vi "GetValue.vi"(0 "reference":refnum<vi>, 1 "Input":string, 3 "error in (no error)":errorcluster) -> (7 "Answer":string, 9 "Found?":bool, 10 "error out":errorcluster)   [LabVIEW 2019]
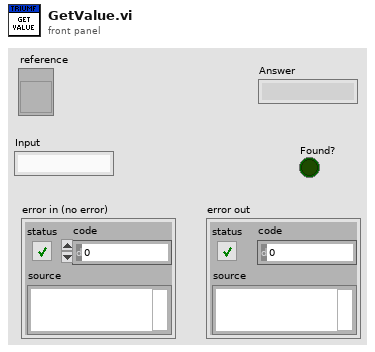
[diagram p1: front panel]
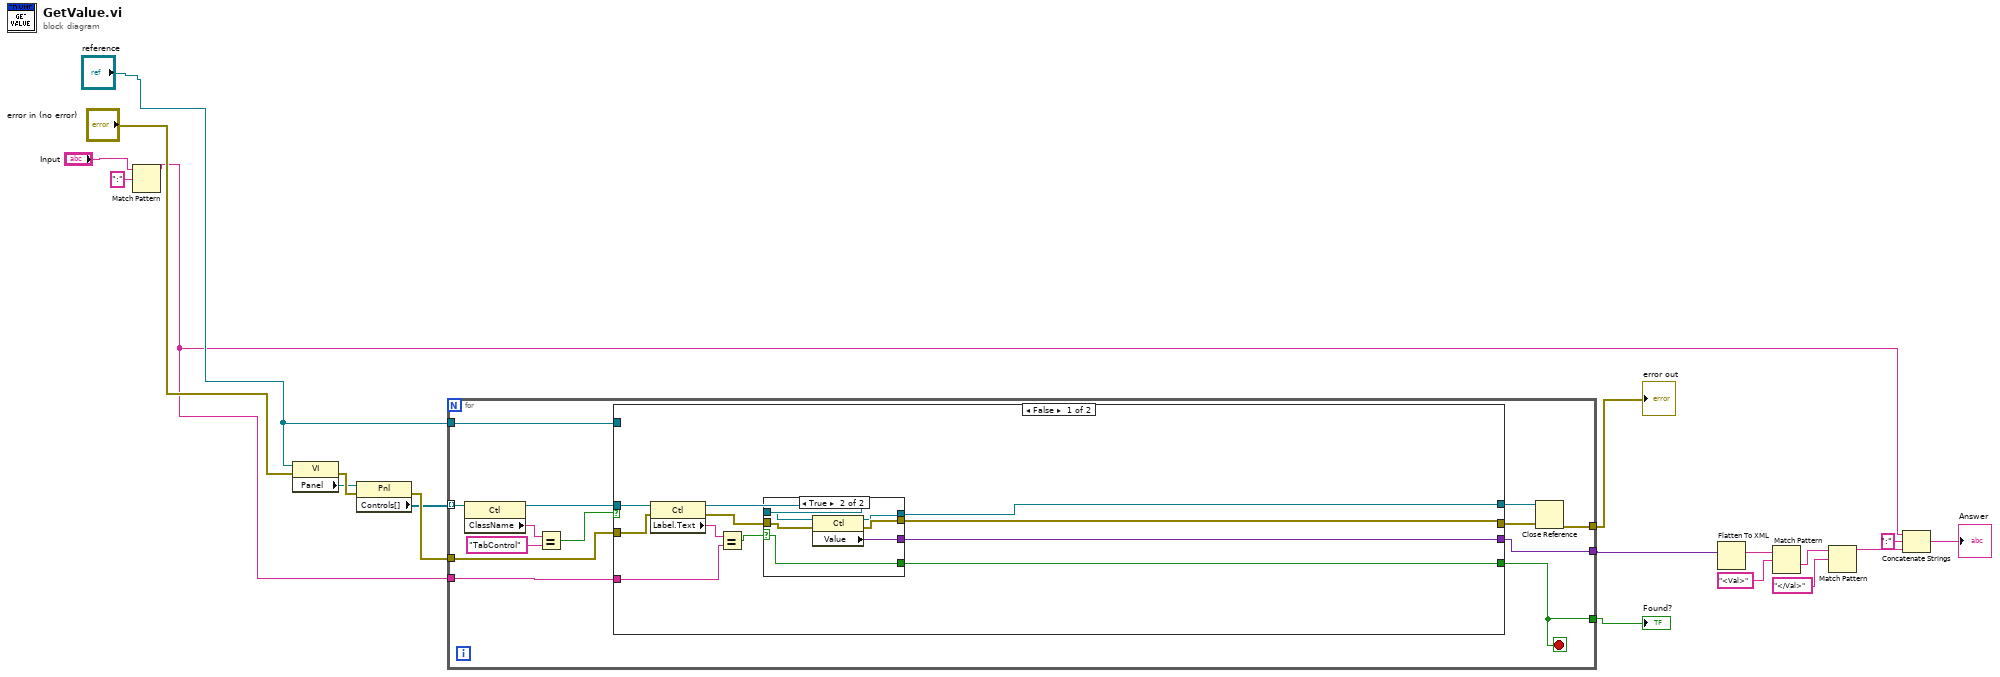
[diagram p0: block diagram]
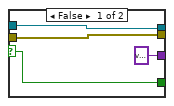
[diagram p2: hidden frame]
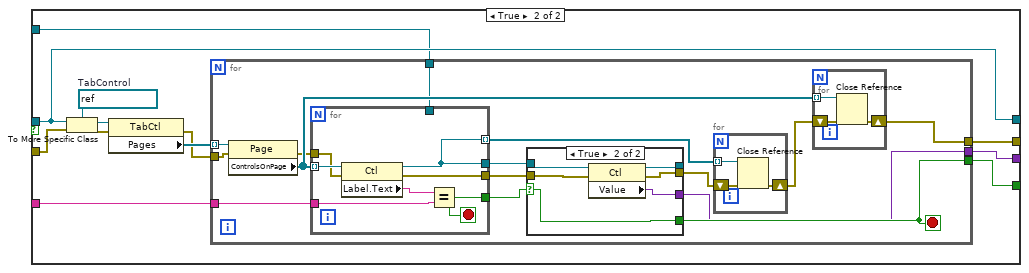
[diagram p3: hidden frame]
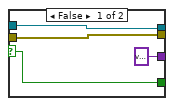
[diagram p4: hidden frame]
diagram:
  n1 = Match Pattern(string="Input", regular expression=":") -> (before substring=w1:string)  [unwired: 1 in, 3 out]
  n2 = property class="VI"(reference="reference", error in="error in (no error)") -> (error out=w14:errorcluster, "Panel"=w13:refnum<vi>)  [unwired: 1 out]
  n3 = property class="Pnl"(reference=w13, error in=w14) -> (error out=w15:errorcluster, "Controls[]"=w12:refnum<vi>[])  [unwired: 1 out]
  n4 = for {
    tunnel: w12 -> [w32] mode=indexing
    tunnel: "reference" -> [w25]
    tunnel: [w26] -> w10
    tunnel: w15 -> [w24]
    tunnel: w1 -> [w22]
    tunnel: [w21] -> w11
    tunnel: [w20] -> w3
    stop <- w21 stop-if-true
    n5 = property class="Ctl"(reference=w32) -> (reference out=w30:refnum<vi>, "ClassName"=w23:string)  [unwired: 1 in, 1 out]
    n6 = Equal?(x=w23, y="TabControl") -> (x = y?=w29:bool)
    n7 = case shown="False" w29 {
      tunnel: w30 -> [w43 w61]
      tunnel: [w35 w62] -> w28
      tunnel: [w36 w61] -> w27
      tunnel: w25 -> [_ w60]
      tunnel: w24 -> [w42 w59]
      tunnel: w22 -> [w40 w56]
      tunnel: [w34 w55] -> w21
      tunnel: [w33 w54] -> w20
      frame False {
        n8 = property class="Ctl"(reference=w43, error in=w42) -> (reference out=w37:refnum<vi>, error out=w38:errorcluster, "Label.Text"=w41:string)
        n9 = Equal?(x=w41, y=w40) -> (x = y?=w39:bool)
        n10 = case shown="True" w39 {
          selector: w39 -> [w45 w53]
          tunnel: [w47 w48] -> w36
          tunnel: w37 -> [w47 w52]
          tunnel: w38 -> [w46 w51]
          tunnel: [w46 w49] -> w35
          tunnel: [w45 w53] -> w34
          tunnel: [variant ("Value") w50] -> w33
          frame False {
          }
          frame True {
            n11 = property class="Ctl"(reference=w52, error in=w51) -> (reference out=w48:refnum<vi>, error out=w49:errorcluster, "Value"=w50:variant)
          }
        }
      }
      frame True {
        w64 = refnum<vi> refnum  # TabControl
        n12 = To More Specific Class(target class=w64, reference=w61, error in=w59) -> (specific class reference=w65:refnum<vi>, error out=w58:errorcluster)
        n13 = property class="TabCtl"(reference=w65, error in=w58) -> (error out=w57:errorcluster, "Pages"=w63:refnum<vi>[])  [unwired: 1 out]
        n14 = for {
          tunnel: w63 -> [w80] mode=indexing
          tunnel: [w78] -> w62
          tunnel: w60 -> [w77]
          tunnel: w57 -> [w76]
          tunnel: w56 -> [w74]
          tunnel: [w70] -> w55
          tunnel: [w66] -> w54
          stop <- w70 stop-if-true
          n15 = property class="Page"(reference=w80, error in=w76) -> (error out=w75:errorcluster, "ControlsOnPage"=w79:refnum<vi>[])  [unwired: 1 out]
          n16 = for {
            tunnel: w79 -> [w103] mode=indexing
            tunnel: [w98] -> w72
            tunnel: w77 -> [_]
            tunnel: w75 -> [w102]
            tunnel: w74 -> [w100]
            tunnel: [w99] -> w71
            tunnel: [w97] -> w69 mode=indexing
            tunnel: [w97] -> w73
            stop <- w99 stop-if-true
            n17 = property class="Ctl"(reference=w103, error in=w102) -> (reference out=w97:refnum<vi>, error out=w98:errorcluster, "Label.Text"=w101:string)
            n18 = Equal?(x=w101, y=w100) -> (x = y?=w99:bool)
          }
          n19 = case shown="True" w71 {
            selector: w71 -> [w85 w89]
            tunnel: [w87 w93] -> _
            tunnel: w73 -> [w87 w92]
            tunnel: w72 -> [w86 w91]
            tunnel: [w86 w90] -> w68
            tunnel: [w85 w89] -> w70
            tunnel: [variant ("Value") w88] -> w66
            frame False {
            }
            frame True {
              n20 = property class="Ctl"(reference=w92, error in=w91) -> (reference out=w93:refnum<vi>, error out=w90:errorcluster, "Value"=w88:variant)
            }
          }
          n21 = for {
            tunnel: w69 -> [w83] mode=indexing
            shift-right: [w82] -> w67
            shift-left: w68 -> [w81]
            n22 = Close Reference(reference=w83, error in (no error)=w81) -> (error out=w82:errorcluster)
          }
          n23 = for {
            tunnel: w79 -> [w96] mode=indexing
            shift-right: [w95] -> w78
            shift-left: w67 -> [w94]
            n24 = Close Reference(reference=w96, error in (no error)=w94) -> (error out=w95:errorcluster)
          }
        }
      }
    }
    n25 = Close Reference(reference=w27, error in (no error)=w28) -> (error out=w26:errorcluster)
  }
  "error out" <- w10
  "Found?" <- w11
  n26 = Flatten To XML(anything=w3) -> (xml string=w8:string)
  n27 = Match Pattern(string=w8, regular expression="<Val>") -> (after substring=w9:string)  [unwired: 1 in, 3 out]
  n28 = Match Pattern(string=w9, regular expression="</Val>") -> (before substring=w4:string)  [unwired: 1 in, 3 out]
  n29 = Concatenate Strings(w1, ":" ("string"), w4) -> (→"Answer":string)
